vi "32xx_Term_Ch.vi"(4 "Msg :Termination Character Enable":bool=TRUE, 6 "Msg :Send End Enable":bool, 7 "Term Ch":string="\r", 8 "error in":errorcluster, 9 "Serial Settings:End Mode for Writes":u16(ring) items=["None", "Last Bit", "TermChar", "Break"], 10 "Serial Settings:End Mode for Reads":u16(ring)=2 items=["None", "Last Bit", "TermChar"], 11 "Visa In":refnum<visa-resource-name>="COM3") -> (0 "error out":errorcluster, 3 "Visa Out":refnum<visa-resource-name>="COM3" caption="Port de sortie")   [LabVIEW 2020]
panel:
  out "Msg Bsd Set:Termination Character":u8=13 format="%x"
  # "Default = \\r"
  # "Default = None"
  # "Default = term Char"
  # "(for Write)"
  # "(for R/W)"
  # "Default = False"
  # "Default = Disable"
  # "© 2008 2020 elc  ALL RIGHTS RESERVED."
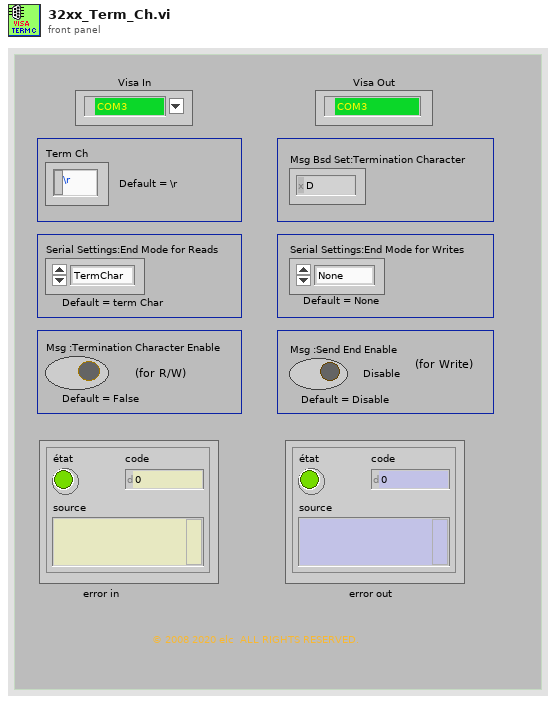
[diagram p1: front panel]
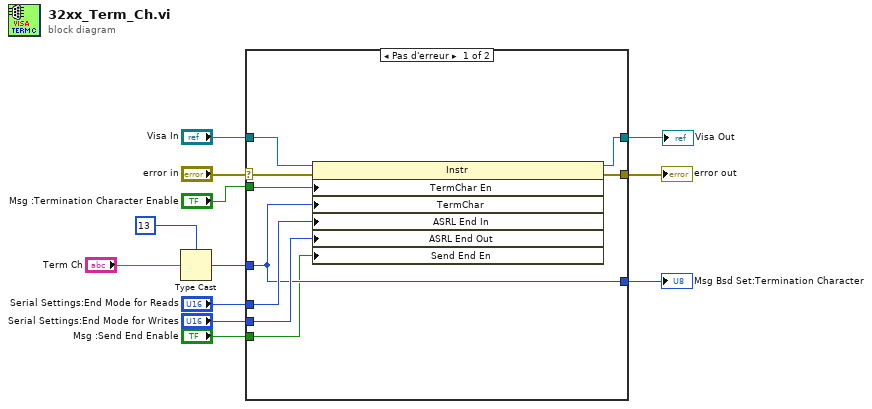
[diagram p0: block diagram]
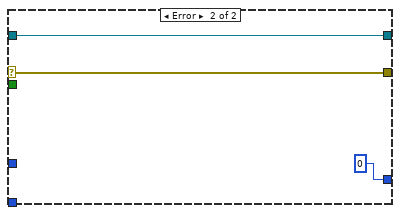
[diagram p2: hidden frame]
diagram:
  n1 = Type Cast(type=u8 13 ("Message Based Settings:Termination Character 2"), x="Term Ch") -> (*(type *) &x=w2:u8)
  n2 = case shown="Pas d'erreur" "error in" {
    selector: "error in" -> [w21 w23]
    tunnel: "Visa In" -> [w20 w24]
    tunnel: [w18 w24] -> w10
    tunnel: [w19 w23] -> w9
    tunnel: "Msg :Send End Enable" -> [w13 _]
    tunnel: "Serial Settings:End Mode for Reads" -> [w17 _]
    tunnel: "Msg :Termination Character Enable" -> [w14 _]
    tunnel: "Serial Settings:End Mode for Writes" -> [w16 _]
    tunnel: w2 -> [w15 _]
    tunnel: [w15 u8 0 ("Message Based Settings:Termination Character 2")] -> w1
    frame No Error {
      n3 = property class="Instr"(reference=w20, error in=w21, "TermChar En"=w14, "TermChar"=w15, "ASRL End In"=w17, "ASRL End Out"=w16, "Send End En"=w13) -> (reference out=w18:refnum<visa-resource-name>, error out=w19:errorcluster)
    }
    frame Error {
    }
  }
  "Visa Out" <- w10
  "error out" <- w9
  "Msg Bsd Set:Termination Character" <- w1
